vi "UserCancel_ErrorHandler.vi"(6 "error in":errorcluster, 8 "Prev Master State Input":T1=enum."Init") -> (0 "error out":errorcluster, 3 "All-Quit":bool, 5 "Next State":T1=enum."Init")   [LabVIEW 2019]
doc: "Resets the CCD camera controller and initializes it with Setup String. The default Setup String is \"ldb,1,16,u,0,225,25,b,1,15;sdu,0,1024,1024;cl0;omrm;sron\". \nError, if no -1, is set as 0 if a serial poll detects an error (bit 15 in status bit set)\n\nSet the CCD Setup String Global variable after the command is complete."
uses:
  LV7/OpticsSS.ctl
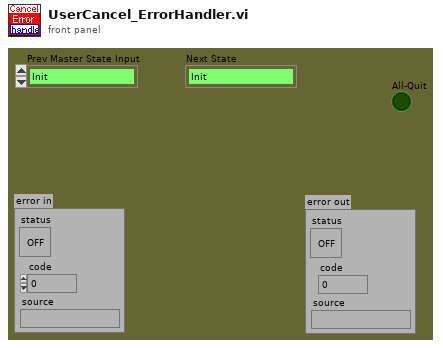
[diagram p1: front panel]
types:
  T1 = typedef "OpticsSS.ctl" = enum16{"_Quit_", "Init", "Ready", "HTL", "CCD_shot", "QueueData", "Error Handler", "HTL Error", "CCD Error", "CCDSetup", "Calibration", "BG_Setup", "HTL Paras Setup"}
  T2 = enum8{"Initialization Error", "Command Error", "Parameter Error", "Overflow Error", "Time-out Error", "Misc Error", "User cancel"}
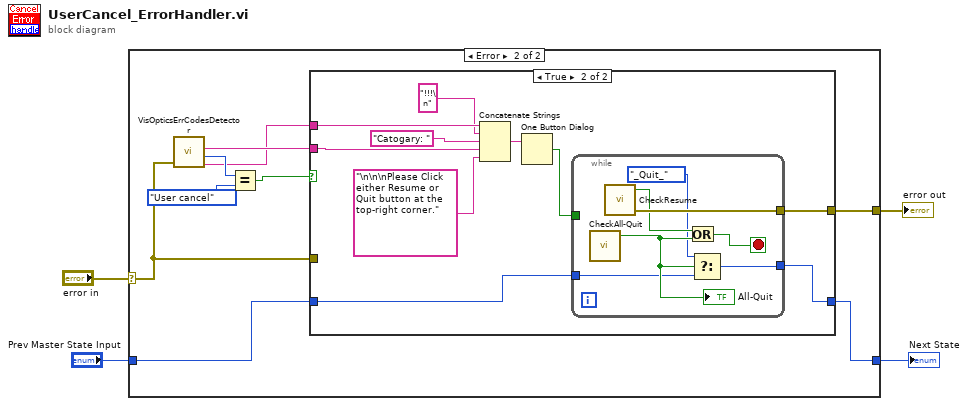
[diagram p0: block diagram]
diagram:
  n1 = case shown="Error" "error in" {
    selector: "error in" -> [w6 w14]
    tunnel: [w6 w15] -> w4
    tunnel: "Prev Master State Input" -> [w5 w8]
    tunnel: [w5 w7] -> w1
    frame No Error {
    }
    frame Error {
      n2 = call "VisOpticsErrCodesDetector.vi"("error in"=w14) -> ("Error Category text"=w13:string, "NHMFL Visible Optics Error Type"=w12:T2, "Error Type text"=w9:string)  [unwired: 2 in, 1 out]
      n3 = Equal?(x=w12, y=T2."User cancel") -> (x = y?=w10:bool)
      n4 = case shown="True" w10 {
        tunnel: [w17 w20] -> w15
        tunnel: w14 -> [w17 _]
        tunnel: w13 -> [_ w24]
        tunnel: w9 -> [_ w27]
        tunnel: w8 -> [w16 w19]
        tunnel: [w16 w18] -> w7
        frame False {
        }
        frame True {
          n5 = Concatenate Strings(w27, "!!!\n" ("string"), "Catogary: " ("string"), w24, "\n\n\nPlease Click either Resume or Quit button at the top-right corner." ("string")) -> (w22:string)
          n6 = One Button Dialog(message=w22) -> (true=w21:bool)  [unwired: 1 in]
          n7 = while {
            tunnel: w21 -> [_]
            tunnel: [w33] -> w20
            tunnel: w19 -> [w29]
            tunnel: [w28] -> w18
            stop <- w34 stop-if-true
            n8 = call "CheckAll-Quit.vi"() -> ("All-Quit"=w31:bool)  [unwired: 3 in]
            "All-Quit" <- w31
            n9 = call "CheckResume.vi"() -> ("Resumed"=w32:bool, "error out"=w33:errorcluster)  [unwired: 2 in]
            n10 = Or(x=w32, y=w31) -> (x .or. y?=w34:bool)
            n11 = Select(t=OpticsSS."_Quit_" ("f"), s=w31, f=w29) -> (s? t:f=w28:T1)
          }
        }
      }
    }
  }
  "error out" <- w4
  "Next State" <- w1
